vi "Destroy.vi"(0 "reference in":refnum<class "Timing.lvclass">, 5 "error in (no error)":errorcluster) -> (14 "reference out":refnum<class "Timing.lvclass">, 19 "error out":errorcluster)   [LabVIEW 2019, in "Timing.lvclass"]
uses:
  Timing.lvclass
  <vilib>/addons/_AddQ/G#Object/G#Object.lvclass
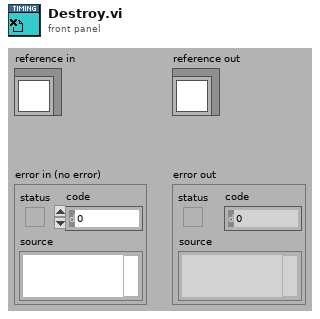
[diagram p1: front panel]
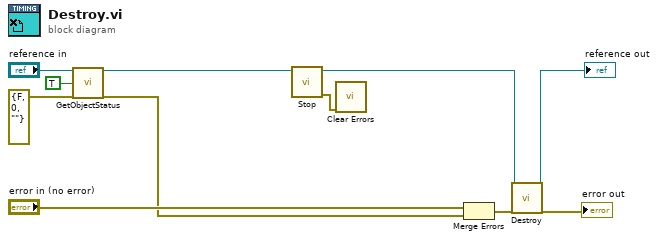
[diagram p0: block diagram]
diagram:
  n1 = call-dynamic "GetObjectStatus.vi"("reference in"="reference in", "simple info (F)"=TRUE ("simple info"), "error in (no error)"=errorcluster {"status"=FALSE, "code"=0, "source"=""}) -> ("reference out"=w3:refnum<class "Timing.lvclass">, "error out"=w4:errorcluster)  [unwired: 5 in, 10 out]
  n2 = call-dynamic "Stop.vi"("reference in"=w3) -> ("error out"=w1:errorcluster, "reference out"=w2:refnum<class "Timing.lvclass">)  [unwired: 9 in]
  n3 = call <vilib>:"Clear Errors.vi"("error in (no error)"=w1) -> ()  [unwired: 5 in, 2 out]
  n4 = Merge Errors("error in (no error)", w4) -> (w10:errorcluster)
  n5 = call-parent "Destroy.vi"("reference in"=w2, "error in (no error)"=w10) -> ("reference out"=→"reference out":refnum<class "Timing.lvclass">, "error out"=→"error out":errorcluster)  [unwired: 16 in]
